vi "Obtain Filtered PPL Class List.vi"(5 "Return all if no filters?(F)":bool, 7 "Force reload?(F)":bool, 8 "error in":errorcluster, 9 "Post-fix filter(\"\")":string, 10 "Contains filter(\"\")":string, 11 "Pre-fix filter(\"\")":string) -> (0 "error out":errorcluster, 2 "PPL Class File Names":string[](array[string]), 3 "PPL Class Paths":path[](array[path]))   [LabVIEW 2020, in "Utility.lvlib"]
doc: "Use this VI to return a subset of the PPL classes. All filters are case independent."
uses:
  Utility.lvlib
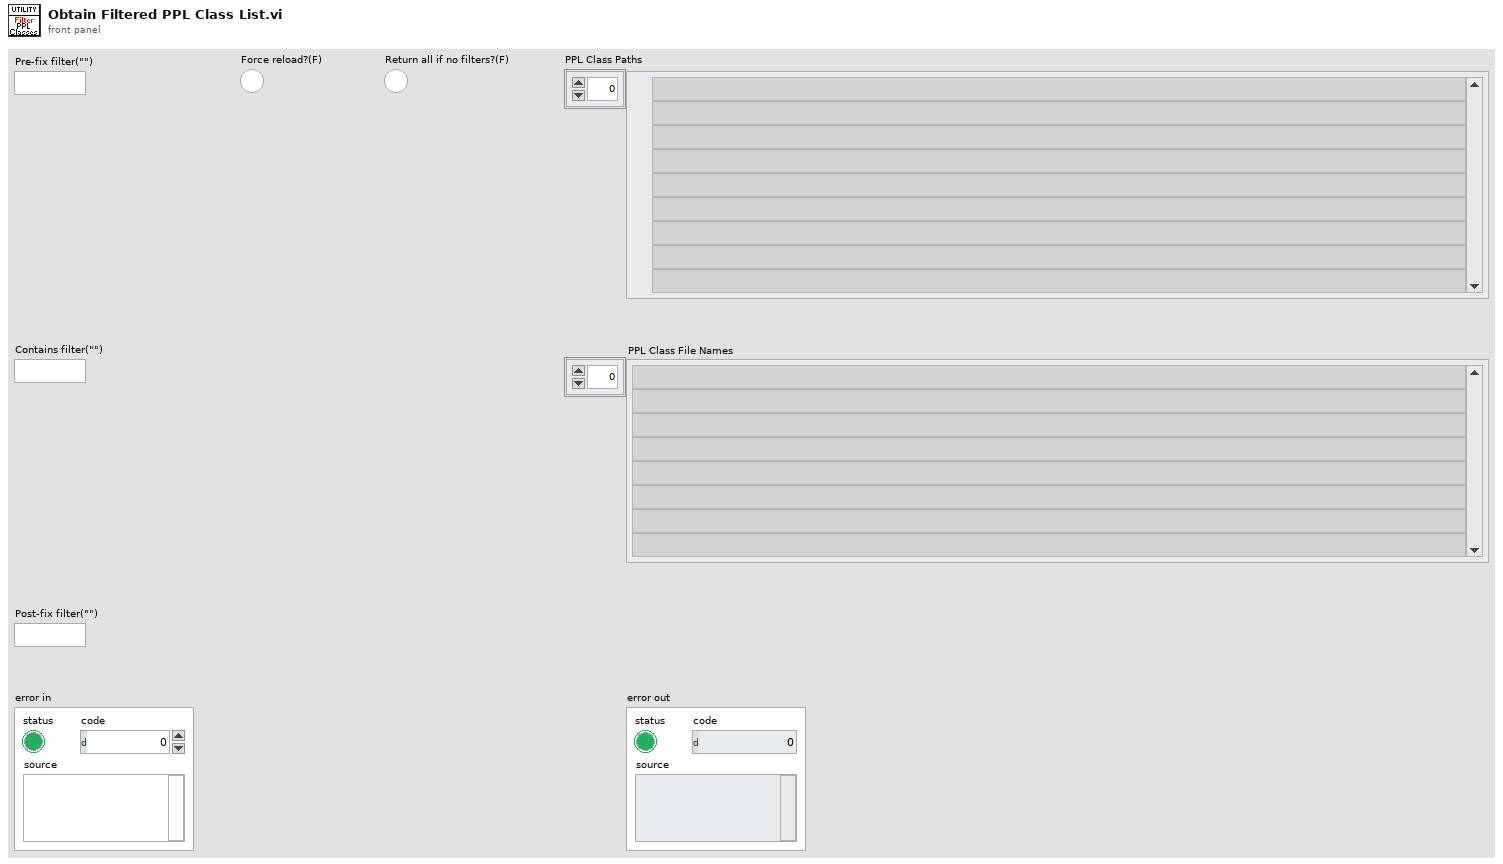
[diagram p1: front panel]
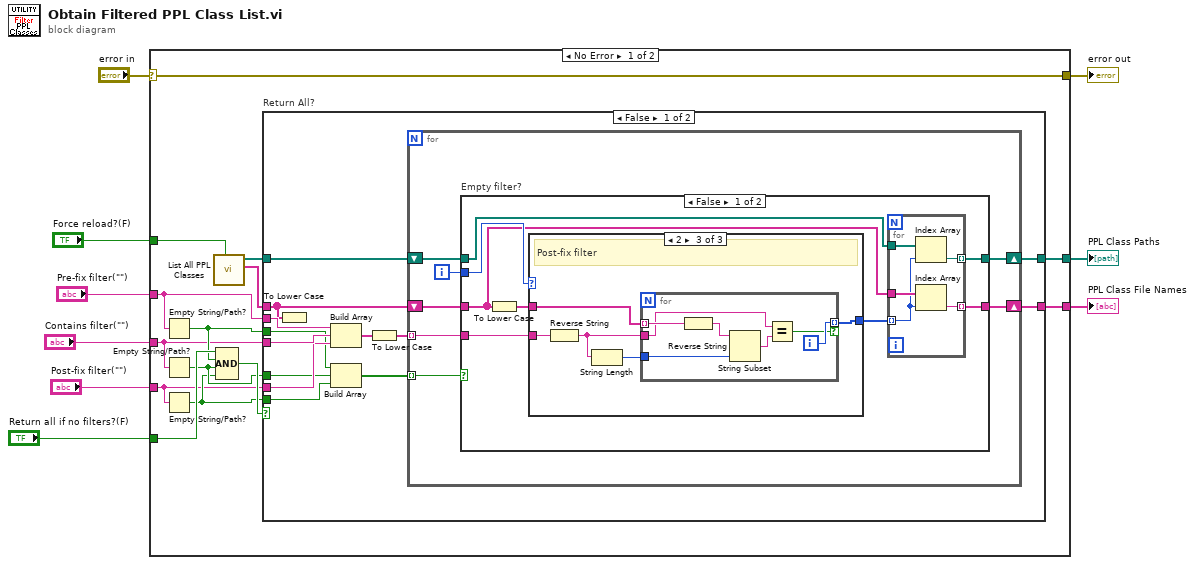
[diagram p0: block diagram]
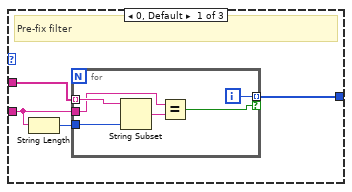
[diagram p2: hidden frame]
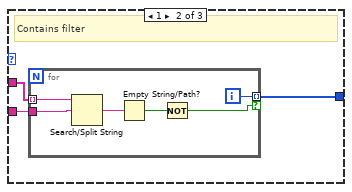
[diagram p3: hidden frame]
diagram:
  n1 = case shown="No Error" "error in" {
    selector: "error in" -> [w10 w92]
    tunnel: "Force reload?(F)" -> [w23 _]
    tunnel: [w18 _] -> w8
    tunnel: [w20 _] -> w7
    tunnel: [w10 w92] -> w5
    tunnel: "Pre-fix filter(\"\")" -> [w15 _]
    tunnel: "Contains filter(\"\")" -> [w13 _]
    tunnel: "Post-fix filter(\"\")" -> [w11 _]
    tunnel: "Return all if no filters?(F)" -> [w22 _]
    frame No Error {
      n2 = Empty String/Path?(string/path=w15) -> (empty?=w16:bool)
      n3 = Empty String/Path?(string/path=w13) -> (empty?=w14:bool)
      n4 = Empty String/Path?(string/path=w11) -> (empty?=w12:bool)
      n5 = call "List All PPL Classes.vi"("Force reload?(F)"=w23) -> ("PPL Class File Names"=w17:string[], "PPL Class Paths"=w19:path[])  [unwired: 9 in]
      n6 = Compound Arithmetic op=AND(w22, w16, w14, w12) -> (w21:bool)
      n7 = case "Return All?" shown="False" w21 {
        tunnel: [w25 w91] -> w20
        tunnel: w19 -> [w27 w91]
        tunnel: [w24 w90] -> w18
        tunnel: w17 -> [w26 w90]
        tunnel: w16 -> [w29 _]
        tunnel: w15 -> [w36 _]
        tunnel: w14 -> [w32 _]
        tunnel: w13 -> [w35 _]
        tunnel: w12 -> [w31 _]
        tunnel: w11 -> [w34 _]
        frame False {
          n8 = To Lower Case(string=w26) -> ()  [unwired: 1 out]
          n9 = Build Array(w36, w35, w34) -> (w33:string[])
          n10 = Build Array(w29, w32, w31) -> (w28:bool[])
          n11 = To Lower Case(string=w33) -> (all lower case string=w30:string[])
          n12 = for {
            tunnel: w30 -> [w37] mode=indexing
            tunnel: w28 -> [w42] mode=indexing
            shift-right: [w41] -> w25
            shift-left: w27 -> [w40]
            shift-right: [w39] -> w24
            shift-left: w26 -> [w38]
            i -> [w43]
            n13 = case "Empty filter?" shown="False" w42 {
              tunnel: w43 -> [w51 _]
              tunnel: [w49 w89] -> w41
              tunnel: w40 -> [w50 w89]
              tunnel: [w48 w88] -> w39
              tunnel: w38 -> [w47 w88]
              tunnel: w37 -> [w45 _]
              frame False {
                n14 = To Lower Case(string=w47) -> (all lower case string=w46:string[])
                n15 = case shown="2" w51 {
                  tunnel: w46 -> [w60 w68 w80]
                  tunnel: w45 -> [w59 w69 w79]
                  tunnel: [w58 w67 w78] -> w44
                  frame 0, Default {
                    # "Pre-fix filter"
                    n16 = String Length(string=w59) -> (length=w57:i32)
                    n17 = for {
                      tunnel: w59 -> [w64]
                      tunnel: w60 -> [w65] mode=indexing
                      tunnel: w57 -> [w66]
                      tunnel: [w62] -> w58 mode=indexing if=w61
                      i -> [w62]
                      n18 = String Subset(string=w65, length (rest)=w66) -> (substring=w63:string)  [unwired: 1 in]
                      n19 = Equal?(x=w64, y=w63) -> (x = y?=w61:bool)
                    }
                  }
                  frame 1 {
                    # "Contains filter"
                    n20 = for {
                      tunnel: w68 -> [w75] mode=indexing
                      tunnel: w69 -> [w74]
                      tunnel: [w71] -> w67 mode=indexing if=w70
                      i -> [w71]
                      n21 = Search/Split String(string=w75, search string/char (-)=w74) -> (match + rest of string=w73:string)  [unwired: 1 in, 2 out]
                      n22 = Empty String/Path?(string/path=w73) -> (empty?=w72:bool)
                      n23 = Not(x=w72) -> (.not. x?=w70:bool)
                    }
                  }
                  frame 2 {
                    # "Post-fix filter"
                    n24 = Reverse String(1:w79) -> (0:w76:string)
                    n25 = String Length(string=w76) -> (length=w77:i32)
                    n26 = for {
                      tunnel: w76 -> [w85]
                      tunnel: w80 -> [w86] mode=indexing
                      tunnel: w77 -> [w87]
                      tunnel: [w83] -> w78 mode=indexing if=w82
                      i -> [w83]
                      n27 = Reverse String(1:w86) -> (0:w81:string)
                      n28 = String Subset(string=w81, length (rest)=w87) -> (substring=w84:string)  [unwired: 1 in]
                      n29 = Equal?(x=w85, y=w84) -> (x = y?=w82:bool)
                    }
                  }
                }
                n30 = for {
                  tunnel: w44 -> [w54] mode=indexing
                  tunnel: w50 -> [w56]
                  tunnel: w47 -> [w55]
                  tunnel: [w53] -> w49 mode=indexing
                  tunnel: [w52] -> w48 mode=indexing
                  n31 = Index Array(array=w56, index=w54) -> (element=w53:path)
                  n32 = Index Array(array=w55, index=w54) -> (element=w52:string)
                }
              }
              frame True {
              }
            }
          }
        }
        frame True {
        }
      }
    }
    frame Error {
    }
  }
  "PPL Class File Names" <- w8
  "PPL Class Paths" <- w7
  "error out" <- w5
